vi "Global Loop.vi"() -> ()   [LabVIEW 2012]
uses:
  <vilib>/Platform/TimedLoop/XDataNode/timing_clust.ctl
  <vilib>/Platform/TimedLoop/XDataNode/nitl_modes.ctl
  <vilib>/Platform/TimedLoop/XDataNode/wakeup.ctl
  Utilities/Robot Parameters/Robot Parameters.vi
  <vilib>/Platform/TimedLoop/XDataNode/XDataNode.xnode
  <vilib>/Platform/TimedLoop/XDataNode/XDNodeRunTimeDep.lvlib
panel:
  in  "stop?":bool
  out "Error Out":errorcluster
  in  "Error In":errorcluster
  out "GPS Waypoint CSV Path":path
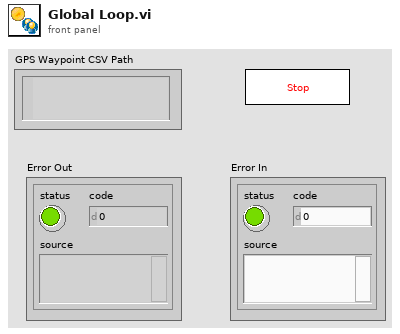
[diagram p1: front panel]
types:
  T1 = cluster{"Latitude":dbl, "Longitude":dbl, "Altitude":dbl, "Velocity, Correction & SET":cluster{"Velocity North":dbl, "Velocity East":dbl, "Velocity Up":dbl, "Ellipsoidal Height":dbl, "GDOP":sgl, "PDOP":sgl, "HDOP":sgl, "VDOP":sgl, "TDOP":sgl, "Horizontal Figure of Merit":u8, "Time Figure of Merit":u8, "Max dGPS Age":sgl, "Extended Navigation Mode":u8, "Antenna Height Adjustment ":dbl, "SET North":i32, "SET East":i32, "SET Up":i32}, "Time":cluster{"GPS Week":u16, "GPS Time of Week":sgl}, "Satellites Used":i32[]}[]
  T2 = cluster{"Latitude":dbl, "Longitude":dbl, "Altitude":dbl, "Velocity, Correction & SET":cluster{"Velocity North":dbl, "Velocity East":dbl, "Velocity Up":dbl, "Ellipsoidal Height":dbl, "GDOP":sgl, "PDOP":sgl, "HDOP":sgl, "VDOP":sgl, "TDOP":sgl, "Horizontal Figure of Merit":u8, "Time Figure of Merit":u8, "Max dGPS Age":sgl, "Extended Navigation Mode":u8, "Antenna Height Adjustment ":dbl, "SET North":i32, "SET East":i32, "SET Up":i32}, "Time":cluster{"GPS Week":u16, "GPS Time of Week":sgl}, "Satellites Used":i32[]}
  T3 = typedef "XDNodeRunTimeDep.lvlib/timing_clust.ctl" = cluster{"Expected End [f-1]":u64, "Actual End [f-1]":u64, "Finished Late? [f-1]":bool, "Expected End [i-1]":u64, "Actual End [i-1]":u64, "Finished Late? [i-1]":bool, "Expected Start [i]":u64, "Actual Start [i]":u64, "Expected Start [f]":u64, "Actual Start [f]":u64, "Source Name":string, "Structure Name":string, "Period":i64, "Deadline":i64, "Offset":i64, "Start":i64, "Priority":i32, "Timeout":i32, "Mode":T4, "Wakeup Reason":T5, "Error":errorcluster, "Source Type":string, "Secondary Source Type":string, "Global End Time":u64, "Global Start Time":u64, "Frame Duration":u64, "Iteration Duration":u64, "Assigned CPU":i32, "I/O Scan Engine Mode":u32}
  T4 = typedef "XDNodeRunTimeDep.lvlib/nitl_modes.ctl" = enum32{"No Change", "Process missed periods, maintain original phase", "Discard missed periods, maintain original phase", "Process missed periods, ignore original phase", "Discard missed periods, ignore original phase"}
  T5 = typedef "XDNodeRunTimeDep.lvlib/wakeup.ctl" = enum32{"Normal", "Aborted", "Asynchronous wakeup", "Timing source error", "Timed loop error", "Timeout"}
  T6 = enum16{"Idle", "Wiimote", "Joypad", "IGVC", "Avoide Objects", "Avoide Lines", "Path Planning", "Heading", "Waypoint"}
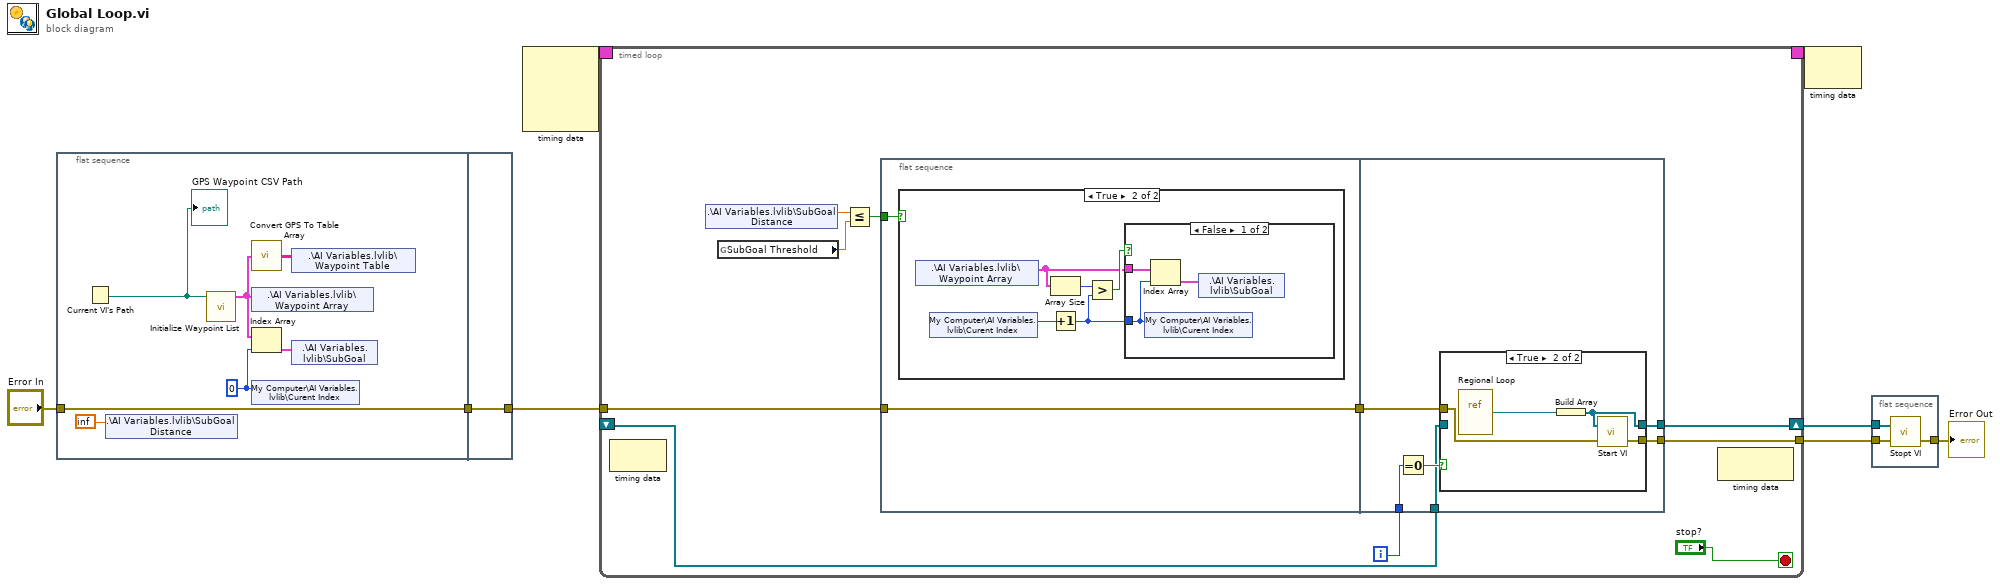
[diagram p0: block diagram]
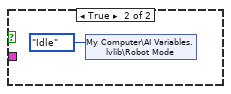
[diagram p3: hidden frame]
diagram:
  n1 = flat-sequence {
    tunnel: "Error In" -> [w15]
    tunnel: [w15] -> w8
    tunnel: [w16] -> w4
    tunnel: w8 -> [w16]
    frame #0 {
      w9 = 0 ("index")
      n2 = Current VI's Path() -> (path=w12:path)
      "GPS Waypoint CSV Path" <- w12
      n3 = shared-variable ".\\AI Variables.lvlib\\SubGoal Distance"(inf) -> ()  [unwired: 1 in, 1 out]
      n4 = call "Initialize Waypoint List.vi"("GPS Waypoint CSV Path"=w12) -> ("Waypoint Array"=w14:T1)  [unwired: 10 in]
      n5 = call "Convert GPS To Table Array.vi"("Waypoint Array In"=w14) -> ("Lat/Long Array Out"=w13:string[][])
      n6 = shared-variable ".\\AI Variables.lvlib\\Waypoint Array"(w14) -> ()  [unwired: 1 in, 1 out]
      n7 = Index Array(array=w14, index=w9) -> (element=w10:T2)
      n8 = shared-variable "My Computer\\AI Variables.lvlib\\Curent Index"(w9) -> ()  [unwired: 1 in, 1 out]
      n9 = shared-variable ".\\AI Variables.lvlib\\Waypoint Table"(w13) -> ()  [unwired: 1 in, 1 out]
      n10 = shared-variable ".\\AI Variables.lvlib\\SubGoal"(w10) -> ()  [unwired: 1 in, 1 out]
    }
    frame #1 {
    }
  }
  n11 = node-c288() -> (w6:T3)  [unwired: 4 in]
  n12 = timed-loop {
    timing: w6 -> [_]
    timing-out: [_] -> w5
    tunnel: w4 -> [w23]
    tunnel: [w22] -> w3
    shift-right: [w24] -> w1
    shift-left: _ -> [w21]
    i -> [w25]
    stop <- "stop?" stop-if-true
    n13 = node-c288() -> ()  [unwired: 1 in, 1 out]
    n14 = shared-variable ".\\AI Variables.lvlib\\SubGoal Distance"() -> (w19:dbl)  [unwired: 1 in, 1 out]
    n15 = global read "Robot Parameters.vi" "SubGoal Threshold"() -> (w18:dbl)
    n16 = Less Or Equal?(x=w19, y=w18) -> (x <= y?=w17:bool)
    n17 = flat-sequence {
      tunnel: w23 -> [w28]
      tunnel: [w28] -> w20
      tunnel: w17 -> [w27]
      tunnel: w25 -> [w42]
      tunnel: [w41] -> w24
      tunnel: [w39] -> w22
      tunnel: w21 -> [w38]
      tunnel: w20 -> [w40]
      frame #0 {
        n18 = case shown="True" w27 {
          frame False {
          }
          frame True {
            n19 = shared-variable ".\\AI Variables.lvlib\\Waypoint Array"() -> (w29:T1)  [unwired: 1 in, 1 out]
            n20 = shared-variable "My Computer\\AI Variables.lvlib\\Curent Index"() -> (w33:i32)  [unwired: 1 in, 1 out]
            n21 = Array Size(array=w29) -> (size(s)=w32:i32)
            n22 = Increment(x=w33) -> (x+1=w30:i32)
            n23 = Greater?(x=w32, y=w30) -> (0:w31:bool)
            n24 = case shown="False" w31 {
              tunnel: w29 -> [w35 _]
              tunnel: w30 -> [w34 _]
              frame False {
                n25 = shared-variable "My Computer\\AI Variables.lvlib\\Curent Index"(w34) -> ()  [unwired: 1 in, 1 out]
                n26 = Index Array(array=w35, index=w34) -> (element=w36:T2)
                n27 = shared-variable ".\\AI Variables.lvlib\\SubGoal"(w36) -> ()  [unwired: 1 in, 1 out]
              }
              frame True {
                n28 = shared-variable "My Computer\\AI Variables.lvlib\\Robot Mode"(T6."Idle" ("Robot Mode")) -> ()  [unwired: 1 in, 1 out]
              }
            }
          }
        }
      }
      frame #1 {
        n29 = Equal To 0?(x=w42) -> (x = 0?=w43:bool)
        n30 = case shown="True" w43 {
          tunnel: [w45 w48] -> w39
          tunnel: [w44 w47] -> w41
          tunnel: w40 -> [w45 w46]
          tunnel: w38 -> [w44 _]
          frame False {
          }
          frame True {
            n31 = vi-ref "Regional Loop.vi"() -> (w49:refnum<vi>)
            n32 = Build Array(w49) -> (w47:refnum<vi>[])
            n33 = call "Start VI.vi"("error in"=w46, "VI refnum"=w47) -> ("error out"=w48:errorcluster)  [unwired: 1 in]
          }
        }
      }
    }
    n34 = node-c288() -> ()  [unwired: 1 in, 1 out]
  }
  n35 = node-c288(w5) -> ()  [unwired: 1 out]
  n36 = flat-sequence {
    tunnel: w3 -> [w54]
    tunnel: [w53] -> w2
    tunnel: w1 -> [w52]
    frame #0 {
      n37 = call "Stopt VI.vi"("error in"=w54, "VI refnum"=w52) -> ("error out"=w53:errorcluster)  [unwired: 1 in]
    }
  }
  "Error Out" <- w2
